vi "mark first stim point.vi"(10 "pixel coordinate":cluster{"X":u32, "Y":u32}, 11 "Image In":T1) -> ()   [LabVIEW 2012]
doc: "SciScan 1.2 160622"
uses:
  <vilib>/vision/Image Controls.llb/IMAQ Image.ctl
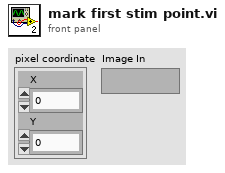
[diagram p1: front panel]
types:
  T1 = typedef "IMAQ Image.ctl" = refnum<image>
  T2 = cluster{"Left":i32, "Top":i32, "Right":i32, "Bottom":i32}
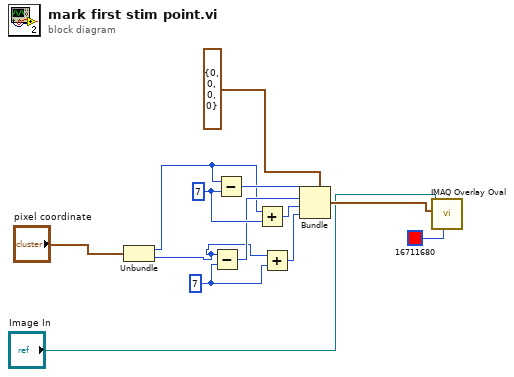
[diagram p0: block diagram]
diagram:
  w8 = 7 ("y")
  w11 = 7 ("y")
  n1 = Unbundle("pixel coordinate") -> ("X"=w5:u32, "Y"=w4:u32)
  n2 = Subtract(x=w4, y=w8) -> (x-y=w7:u32)
  n3 = Subtract(x=w5, y=w11) -> (x-y=w10:u32)
  n4 = Add(x=w5, y=w11) -> (x+y=w12:u32)
  n5 = Add(x=w4, y=w8) -> (x+y=w9:u32)
  n6 = Bundle(cluster=T2 {"Left"=0, "Top"=0, "Right"=0, "Bottom"=0} ("Bounding Rectangle"), "Left"=w10, "Top"=w7, "Right"=w12, "Bottom"=w9) -> (w3:T2)
  n7 = call "IMAQ Overlay Oval"("Color"=u32 16711680, "Bounding Rectangle"=w3, "Image"="Image In") -> ()  [unwired: 7 in, 2 out]
